vi "TyrMt.vi"() -> ()   [LabVIEW 2011]
uses:
  <vilib>/Instr/_visa.llb/VISA Configure Serial Port (Instr).vi
panel:
  in  "VISA resource name":refnum<visa-resource-name>
  in  "Path":path=path "/Users/Optimus/Dropbox/Documents/My_SeniorDesign/controls/"
  out "?":bool
  in  "Data Switch":bool
  in  "stop":bool
  # "CONNECTION INFORMATION"
  # "READ IMU DATA"
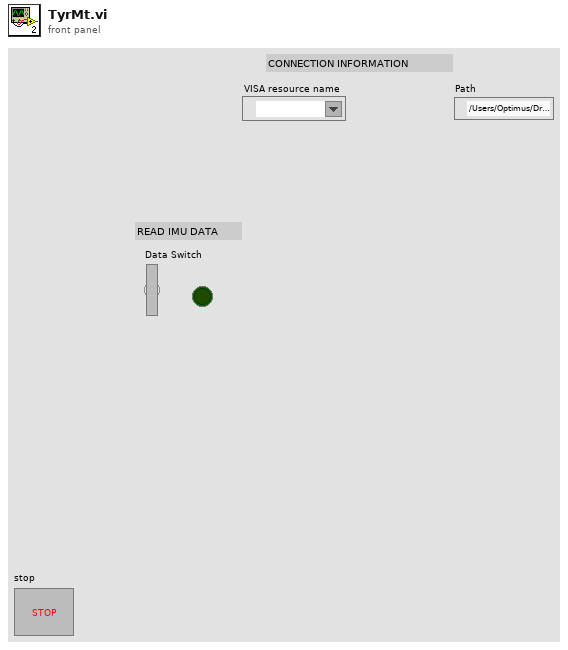
[diagram p1: front panel]
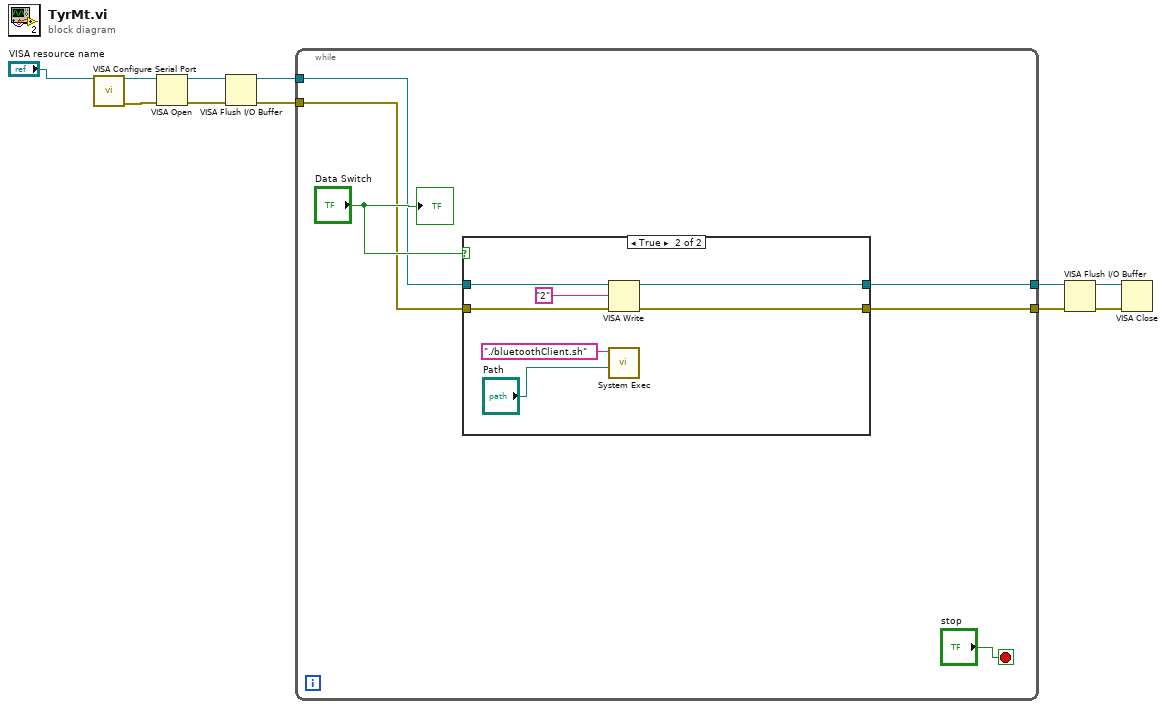
[diagram p0: block diagram]
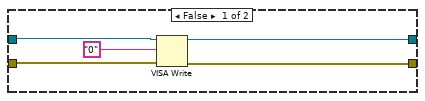
[diagram p2: hidden frame]
diagram:
  n1 = call-poly "VISA Configure Serial Port"("VISA resource name"="VISA resource name") -> ("VISA resource name out"=w5:refnum<visa-resource-name>, "error out"=w4:errorcluster)  [unwired: 13 in]
  n2 = VISA Open(error in (no error)=w4, VISA resource name=w5) -> (VISA resource name=w3:refnum<visa-resource-name>, error out=w2:errorcluster)  [unwired: 3 in]
  n3 = VISA Flush I/O Buffer(VISA resource name=w3, error in (no error)=w2) -> (VISA resource name out=w11:refnum<visa-resource-name>, error out=w10:errorcluster)  [unwired: 1 in]
  n4 = while {
    tunnel: w11 -> [w14]
    tunnel: w10 -> [w15]
    tunnel: [w12] -> w8
    tunnel: [w13] -> w9
    stop <- "stop" stop-if-true
    n5 = case shown="True" "Data Switch" {
      tunnel: w15 -> [w18 w29]
      tunnel: w14 -> [w19 w28]
      tunnel: [w21 w27] -> w12
      tunnel: [w20 w26] -> w13
      frame False {
        n6 = VISA Write(VISA resource name=w19, write buffer="0", error in (no error)=w18) -> (VISA resource name out=w21:refnum<visa-resource-name>, error out=w20:errorcluster)  [unwired: 1 out]
      }
      frame True {
        n7 = VISA Write(VISA resource name=w28, write buffer="2", error in (no error)=w29) -> (VISA resource name out=w27:refnum<visa-resource-name>, error out=w26:errorcluster)  [unwired: 1 out]
        n8 = call <vilib>:"System Exec.vi"("working directory"="Path", "command line"="./bluetoothClient.sh") -> ()  [unwired: 6 in, 4 out]
      }
    }
    "?" <- "Data Switch"
  }
  n9 = VISA Flush I/O Buffer(VISA resource name=w8, error in (no error)=w9) -> (VISA resource name out=w6:refnum<visa-resource-name>, error out=w7:errorcluster)  [unwired: 1 in]
  n10 = VISA Close(VISA resource name=w6, error in (no error)=w7) -> ()  [unwired: 1 out]
